vi "Digilens DLP Gen2 UI .vi"(11 "TopLevel In":refnum<class "TopLevel.lvclass">) -> (3 "TopLevel Out":refnum<class "TopLevel.lvclass">)   [LabVIEW 2022 SP3, in "TopLevel.lvclass"] (continued)
              disable-tunnel: ICP2-DO_Channel_Names."Recirc Pump On - R2" ("DO Channel") -> [w2353 w2369]
              disable-tunnel: w2344 -> [w2352 _]
              disable-tunnel: [w2351 w2354] -> w2343
              disable-tunnel: w2342 -> [w2350 w2370]
              disable-tunnel: "Recirc Pump On - R2" -> [w2349 w2356]
              disable-tunnel: w2340 -> [_ w2368]
              frame Disabled {
                n801 = call-dynamic "Set ICP2-DO Changed bit.vi"("error in (no error)"=w2350, "Value"=w2349, "DO Channel"=w2353, "IO in"=w2352) -> ("error out"=w2351:errorcluster)  [unwired: 6 in, 1 out]
              }
              frame Enabled {
                n802 = Format Into String(format string="%s", w2369) -> (resulting string=w2372:string)  [unwired: 2 in, 1 out]
                n803 = call "Set DO State (manual mode).vi"("error in (no error)"=w2370, "State"=w2356, "DO IOName"=w2372, "DAQ"=w2368) -> ("error out"=w2355:errorcluster, "DAQ"=w2357:refnum<class "DAQ.lvclass">)  [unwired: 6 in]
                n804 = Format Into String(format string="%s", error in=w2355, ICP2-DO_Channel_Names."SW_LED - Ink Valve - R2" ("DO Channel")) -> (resulting string=w2367:string, error out=w2364:errorcluster)  [unwired: 1 in]
                n805 = call "Set DO State (automation mode).vi"("error in (no error)"=w2364, "State"=w2356, "DO IOName"=w2367, "DAQ"=w2357) -> ("error out"=w2358:errorcluster, "DAQ"=w2360:refnum<class "DAQ.lvclass">)  [unwired: 6 in]
                n806 = Format Into String(format string="%s", error in=w2358, ICP2-DO_Channel_Names."Ink Flow Valve Open - R2" ("DO Channel")) -> (resulting string=w2361:string, error out=w2363:errorcluster)  [unwired: 1 in]
                n807 = call "Set DO State (automation mode).vi"("error in (no error)"=w2363, "State"=w2356, "DO IOName"=w2361, "DAQ"=w2360) -> ("error out"=w2354:errorcluster)  [unwired: 6 in, 1 out]
              }
            }
          }
          event "Recirc Pump On - R3": Value Change {
            n808 = event-data() -> ()  [unwired: 1 in, 6 out]
            n809 = Unbundle By Name(w2378) -> ("DAQ"=w2373:refnum<class "DAQ.lvclass">, "IO"=w2377:refnum<class "IO.lvclass">)
            n810 = disable-structure shown="Enabled" {
              disable-tunnel: ICP2-DO_Channel_Names."Recirc Pump On - R3" ("DO Channel") -> [w2386 w2401]
              disable-tunnel: w2377 -> [w2385 _]
              disable-tunnel: [w2384 w2387] -> w2376
              disable-tunnel: w2375 -> [w2383 w2403]
              disable-tunnel: "Recirc Pump On - R3" -> [w2382 w2389]
              disable-tunnel: w2373 -> [_ w2402]
              frame Disabled {
                n811 = call-dynamic "Set ICP2-DO Changed bit.vi"("error in (no error)"=w2383, "Value"=w2382, "DO Channel"=w2386, "IO in"=w2385) -> ("error out"=w2384:errorcluster)  [unwired: 6 in, 1 out]
              }
              frame Enabled {
                n812 = Format Into String(format string="%s", w2401) -> (resulting string=w2405:string)  [unwired: 2 in, 1 out]
                n813 = call "Set DO State (manual mode).vi"("error in (no error)"=w2403, "State"=w2389, "DO IOName"=w2405, "DAQ"=w2402) -> ("error out"=w2388:errorcluster, "DAQ"=w2390:refnum<class "DAQ.lvclass">)  [unwired: 6 in]
                n814 = Format Into String(format string="%s", error in=w2388, ICP2-DO_Channel_Names."SW_LED - Ink Valve - R3" ("DO Channel")) -> (resulting string=w2400:string, error out=w2397:errorcluster)  [unwired: 1 in]
                n815 = call "Set DO State (automation mode).vi"("error in (no error)"=w2397, "State"=w2389, "DO IOName"=w2400, "DAQ"=w2390) -> ("error out"=w2391:errorcluster, "DAQ"=w2393:refnum<class "DAQ.lvclass">)  [unwired: 6 in]
                n816 = Format Into String(format string="%s", error in=w2391, ICP2-DO_Channel_Names."Ink Flow Valve Open - R3" ("DO Channel")) -> (resulting string=w2394:string, error out=w2396:errorcluster)  [unwired: 1 in]
                n817 = call "Set DO State (automation mode).vi"("error in (no error)"=w2396, "State"=w2389, "DO IOName"=w2394, "DAQ"=w2393) -> ("error out"=w2387:errorcluster)  [unwired: 6 in, 1 out]
              }
            }
          }
          event "Recirc Pump On - R4": Value Change {
            n818 = event-data() -> ()  [unwired: 1 in, 6 out]
            n819 = Unbundle By Name(w2411) -> ("DAQ"=w2406:refnum<class "DAQ.lvclass">, "IO"=w2410:refnum<class "IO.lvclass">)
            n820 = disable-structure shown="Enabled" {
              disable-tunnel: ICP2-DO_Channel_Names."Recirc Pump On - R4" ("DO Channel") -> [w2419 w2434]
              disable-tunnel: w2410 -> [w2418 _]
              disable-tunnel: [w2417 w2420] -> w2409
              disable-tunnel: w2408 -> [w2416 w2436]
              disable-tunnel: "Recirc Pump On - R4" -> [w2415 w2421]
              disable-tunnel: w2406 -> [_ w2435]
              frame Disabled {
                n821 = call-dynamic "Set ICP2-DO Changed bit.vi"("error in (no error)"=w2416, "Value"=w2415, "DO Channel"=w2419, "IO in"=w2418) -> ("error out"=w2417:errorcluster)  [unwired: 6 in, 1 out]
              }
              frame Enabled {
                n822 = Format Into String(format string="%s", w2434) -> (resulting string=w2438:string)  [unwired: 2 in, 1 out]
                n823 = call "Set DO State (manual mode).vi"("error in (no error)"=w2436, "State"=w2421, "DO IOName"=w2438, "DAQ"=w2435) -> ("error out"=w2422:errorcluster, "DAQ"=w2423:refnum<class "DAQ.lvclass">)  [unwired: 6 in]
                n824 = Format Into String(format string="%s", error in=w2422, ICP2-DO_Channel_Names."SW_LED - Ink Valve - R4" ("DO Channel")) -> (resulting string=w2433:string, error out=w2430:errorcluster)  [unwired: 1 in]
                n825 = call "Set DO State (automation mode).vi"("error in (no error)"=w2430, "State"=w2421, "DO IOName"=w2433, "DAQ"=w2423) -> ("error out"=w2424:errorcluster, "DAQ"=w2426:refnum<class "DAQ.lvclass">)  [unwired: 6 in]
                n826 = Format Into String(format string="%s", error in=w2424, ICP2-DO_Channel_Names."Ink Flow Valve Open - R4" ("DO Channel")) -> (resulting string=w2427:string, error out=w2429:errorcluster)  [unwired: 1 in]
                n827 = call "Set DO State (automation mode).vi"("error in (no error)"=w2429, "State"=w2421, "DO IOName"=w2427, "DAQ"=w2426) -> ("error out"=w2420:errorcluster)  [unwired: 6 in, 1 out]
              }
            }
          }
          event "Recirc Pump On - R5": Value Change {
            n828 = event-data() -> ()  [unwired: 1 in, 6 out]
            n829 = Unbundle By Name(w2444) -> ("DAQ"=w2439:refnum<class "DAQ.lvclass">, "IO"=w2443:refnum<class "IO.lvclass">)
            n830 = disable-structure shown="Enabled" {
              disable-tunnel: ICP2-DO_Channel_Names."Recirc Pump On - R5" ("DO Channel") -> [w2452 w2468]
              disable-tunnel: w2443 -> [w2451 _]
              disable-tunnel: [w2450 w2453] -> w2442
              disable-tunnel: w2441 -> [w2449 w2469]
              disable-tunnel: "Recirc Pump On - R5" -> [w2448 w2455]
              disable-tunnel: w2439 -> [_ w2467]
              frame Disabled {
                n831 = call-dynamic "Set ICP2-DO Changed bit.vi"("error in (no error)"=w2449, "Value"=w2448, "DO Channel"=w2452, "IO in"=w2451) -> ("error out"=w2450:errorcluster)  [unwired: 6 in, 1 out]
              }
              frame Enabled {
                n832 = Format Into String(format string="%s", w2468) -> (resulting string=w2471:string)  [unwired: 2 in, 1 out]
                n833 = call "Set DO State (manual mode).vi"("error in (no error)"=w2469, "State"=w2455, "DO IOName"=w2471, "DAQ"=w2467) -> ("error out"=w2454:errorcluster, "DAQ"=w2456:refnum<class "DAQ.lvclass">)  [unwired: 6 in]
                n834 = Format Into String(format string="%s", error in=w2454, ICP2-DO_Channel_Names."SW_LED - Ink Valve - R5" ("DO Channel")) -> (resulting string=w2466:string, error out=w2463:errorcluster)  [unwired: 1 in]
                n835 = call "Set DO State (automation mode).vi"("error in (no error)"=w2463, "State"=w2455, "DO IOName"=w2466, "DAQ"=w2456) -> ("error out"=w2457:errorcluster, "DAQ"=w2459:refnum<class "DAQ.lvclass">)  [unwired: 6 in]
                n836 = Format Into String(format string="%s", error in=w2457, ICP2-DO_Channel_Names."Ink Flow Valve Open - R5" ("DO Channel")) -> (resulting string=w2460:string, error out=w2462:errorcluster)  [unwired: 1 in]
                n837 = call "Set DO State (automation mode).vi"("error in (no error)"=w2462, "State"=w2455, "DO IOName"=w2460, "DAQ"=w2459) -> ("error out"=w2453:errorcluster)  [unwired: 6 in, 1 out]
              }
            }
          }
          event "Recirc Pump On - R6": Value Change {
            n838 = event-data() -> ()  [unwired: 1 in, 6 out]
            n839 = Unbundle By Name(w2477) -> ("DAQ"=w2472:refnum<class "DAQ.lvclass">, "IO"=w2476:refnum<class "IO.lvclass">)
            n840 = disable-structure shown="Enabled" {
              disable-tunnel: ICP2-DO_Channel_Names."Recirc Pump On - R6" ("DO Channel") -> [w2485 w2500]
              disable-tunnel: w2476 -> [w2484 _]
              disable-tunnel: [w2483 w2487] -> w2475
              disable-tunnel: w2474 -> [w2482 w2502]
              disable-tunnel: "Recirc Pump On - R6" -> [w2481 w2486]
              disable-tunnel: w2472 -> [_ w2501]
              frame Disabled {
                n841 = call-dynamic "Set ICP2-DO Changed bit.vi"("error in (no error)"=w2482, "Value"=w2481, "DO Channel"=w2485, "IO in"=w2484) -> ("error out"=w2483:errorcluster)  [unwired: 6 in, 1 out]
              }
              frame Enabled {
                n842 = Format Into String(format string="%s", w2500) -> (resulting string=w2504:string)  [unwired: 2 in, 1 out]
                n843 = call "Set DO State (manual mode).vi"("error in (no error)"=w2502, "State"=w2486, "DO IOName"=w2504, "DAQ"=w2501) -> ("error out"=w2488:errorcluster, "DAQ"=w2489:refnum<class "DAQ.lvclass">)  [unwired: 6 in]
                n844 = Format Into String(format string="%s", error in=w2488, ICP2-DO_Channel_Names."SW_LED - Ink Valve - R6" ("DO Channel")) -> (resulting string=w2499:string, error out=w2496:errorcluster)  [unwired: 1 in]
                n845 = call "Set DO State (automation mode).vi"("error in (no error)"=w2496, "State"=w2486, "DO IOName"=w2499, "DAQ"=w2489) -> ("error out"=w2490:errorcluster, "DAQ"=w2492:refnum<class "DAQ.lvclass">)  [unwired: 6 in]
                n846 = Format Into String(format string="%s", error in=w2490, ICP2-DO_Channel_Names."Ink Flow Valve Open - R6" ("DO Channel")) -> (resulting string=w2493:string, error out=w2495:errorcluster)  [unwired: 1 in]
                n847 = call "Set DO State (automation mode).vi"("error in (no error)"=w2495, "State"=w2486, "DO IOName"=w2493, "DAQ"=w2492) -> ("error out"=w2487:errorcluster)  [unwired: 6 in, 1 out]
              }
            }
          }
          event "Meniscus Pressure Reg PWR - R1": Value Change {
            n848 = event-data() -> ()  [unwired: 1 in, 6 out]
            n849 = Unbundle By Name(w2510) -> ("DAQ"=w2505:refnum<class "DAQ.lvclass">, "IO"=w2509:refnum<class "IO.lvclass">)
            n850 = disable-structure shown="Enabled" {
              disable-tunnel: ICP1-D0_Channel_Names."Meniscus Pressure Reg PWR - R1" ("DO Channel") -> [w2518 w2520]
              disable-tunnel: w2509 -> [w2517 _]
              disable-tunnel: [w2516 w2522] -> w2508
              disable-tunnel: w2507 -> [w2515 w2523]
              disable-tunnel: "Meniscus Pressure Reg PWR - R1" -> [w2514 w2521]
              disable-tunnel: w2505 -> [_ w2519]
              frame Disabled {
                n851 = call-dynamic "Set ICP1-DO Changed bit.vi"("error in (no error)"=w2515, "Value"=w2514, "DO Channel"=w2518, "IO in"=w2517) -> ("error out"=w2516:errorcluster)  [unwired: 6 in, 1 out]
              }
              frame Enabled {
                n852 = Format Into String(format string="%s", w2520) -> (resulting string=w2525:string)  [unwired: 2 in, 1 out]
                n853 = call "Set DO State (manual mode).vi"("error in (no error)"=w2523, "State"=w2521, "DO IOName"=w2525, "DAQ"=w2519) -> ("error out"=w2522:errorcluster)  [unwired: 6 in, 1 out]
              }
            }
          }
          event "Meniscus Pressure Reg PWR - R2": Value Change {
            n854 = event-data() -> ()  [unwired: 1 in, 6 out]
            n855 = Unbundle By Name(w2531) -> ("DAQ"=w2526:refnum<class "DAQ.lvclass">, "IO"=w2530:refnum<class "IO.lvclass">)
            n856 = disable-structure shown="Enabled" {
              disable-tunnel: ICP1-D0_Channel_Names."Meniscus Pressure Reg PWR - R2" ("DO Channel") -> [w2539 w2542]
              disable-tunnel: w2530 -> [w2538 _]
              disable-tunnel: [w2537 w2540] -> w2529
              disable-tunnel: w2528 -> [w2536 w2541]
              disable-tunnel: "Meniscus Pressure Reg PWR - R2" -> [w2535 w2544]
              disable-tunnel: w2526 -> [_ w2543]
              frame Disabled {
                n857 = call-dynamic "Set ICP1-DO Changed bit.vi"("error in (no error)"=w2536, "Value"=w2535, "DO Channel"=w2539, "IO in"=w2538) -> ("error out"=w2537:errorcluster)  [unwired: 6 in, 1 out]
              }
              frame Enabled {
                n858 = Format Into String(format string="%s", w2542) -> (resulting string=w2546:string)  [unwired: 2 in, 1 out]
                n859 = call "Set DO State (manual mode).vi"("error in (no error)"=w2541, "State"=w2544, "DO IOName"=w2546, "DAQ"=w2543) -> ("error out"=w2540:errorcluster)  [unwired: 6 in, 1 out]
              }
            }
          }
          event "Meniscus Pressure Reg PWR - R3": Value Change {
            n860 = event-data() -> ()  [unwired: 1 in, 6 out]
            n861 = Unbundle By Name(w2552) -> ("DAQ"=w2547:refnum<class "DAQ.lvclass">, "IO"=w2551:refnum<class "IO.lvclass">)
            n862 = disable-structure shown="Enabled" {
              disable-tunnel: ICP1-D0_Channel_Names."Meniscus Pressure Reg PWR - R3" ("DO Channel") -> [w2560 w2561]
              disable-tunnel: w2551 -> [w2559 _]
              disable-tunnel: [w2558 w2563] -> w2550
              disable-tunnel: w2549 -> [w2557 w2564]
              disable-tunnel: "Meniscus Pressure Reg PWR - R3" -> [w2556 w2565]
              disable-tunnel: w2547 -> [_ w2562]
              frame Disabled {
                n863 = call-dynamic "Set ICP1-DO Changed bit.vi"("error in (no error)"=w2557, "Value"=w2556, "DO Channel"=w2560, "IO in"=w2559) -> ("error out"=w2558:errorcluster)  [unwired: 6 in, 1 out]
              }
              frame Enabled {
                n864 = Format Into String(format string="%s", w2561) -> (resulting string=w2567:string)  [unwired: 2 in, 1 out]
                n865 = call "Set DO State (manual mode).vi"("error in (no error)"=w2564, "State"=w2565, "DO IOName"=w2567, "DAQ"=w2562) -> ("error out"=w2563:errorcluster)  [unwired: 6 in, 1 out]
              }
            }
          }
          event "Meniscus Pressure Reg PWR - R4": Value Change {
            n866 = event-data() -> ()  [unwired: 1 in, 6 out]
            n867 = Unbundle By Name(w2573) -> ("DAQ"=w2568:refnum<class "DAQ.lvclass">, "IO"=w2572:refnum<class "IO.lvclass">)
            n868 = disable-structure shown="Enabled" {
              disable-tunnel: ICP1-D0_Channel_Names."Meniscus Pressure Reg PWR - R4" ("DO Channel") -> [w2581 w2583]
              disable-tunnel: w2572 -> [w2580 _]
              disable-tunnel: [w2579 w2585] -> w2571
              disable-tunnel: w2570 -> [w2578 w2586]
              disable-tunnel: "Meniscus Pressure Reg PWR - R4" -> [w2577 w2584]
              disable-tunnel: w2568 -> [_ w2582]
              frame Disabled {
                n869 = call-dynamic "Set ICP1-DO Changed bit.vi"("error in (no error)"=w2578, "Value"=w2577, "DO Channel"=w2581, "IO in"=w2580) -> ("error out"=w2579:errorcluster)  [unwired: 6 in, 1 out]
              }
              frame Enabled {
                n870 = Format Into String(format string="%s", w2583) -> (resulting string=w2588:string)  [unwired: 2 in, 1 out]
                n871 = call "Set DO State (manual mode).vi"("error in (no error)"=w2586, "State"=w2584, "DO IOName"=w2588, "DAQ"=w2582) -> ("error out"=w2585:errorcluster)  [unwired: 6 in, 1 out]
              }
            }
          }
          event "Meniscus Pressure Reg PWR - R5": Value Change {
            n872 = event-data() -> ()  [unwired: 1 in, 6 out]
            n873 = Unbundle By Name(w2594) -> ("DAQ"=w2589:refnum<class "DAQ.lvclass">, "IO"=w2593:refnum<class "IO.lvclass">)
            n874 = disable-structure shown="Enabled" {
              disable-tunnel: ICP1-D0_Channel_Names."Meniscus Pressure Reg PWR - R5" ("DO Channel") -> [w2602 w2603]
              disable-tunnel: w2593 -> [w2601 _]
              disable-tunnel: [w2600 w2605] -> w2592
              disable-tunnel: w2591 -> [w2599 w2606]
              disable-tunnel: "Meniscus Pressure Reg PWR - R5" -> [w2598 w2607]
              disable-tunnel: w2589 -> [_ w2604]
              frame Disabled {
                n875 = call-dynamic "Set ICP1-DO Changed bit.vi"("error in (no error)"=w2599, "Value"=w2598, "DO Channel"=w2602, "IO in"=w2601) -> ("error out"=w2600:errorcluster)  [unwired: 6 in, 1 out]
              }
              frame Enabled {
                n876 = Format Into String(format string="%s", w2603) -> (resulting string=w2609:string)  [unwired: 2 in, 1 out]
                n877 = call "Set DO State (manual mode).vi"("error in (no error)"=w2606, "State"=w2607, "DO IOName"=w2609, "DAQ"=w2604) -> ("error out"=w2605:errorcluster)  [unwired: 6 in, 1 out]
              }
            }
          }
          event "Meniscus Pressure Reg PWR - R6": Value Change {
            n878 = event-data() -> ()  [unwired: 1 in, 6 out]
            n879 = Unbundle By Name(w2615) -> ("DAQ"=w2610:refnum<class "DAQ.lvclass">, "IO"=w2614:refnum<class "IO.lvclass">)
            n880 = disable-structure shown="Enabled" {
              disable-tunnel: ICP1-D0_Channel_Names."Meniscus Pressure Reg PWR - R6" ("DO Channel") -> [w2623 w2624]
              disable-tunnel: w2614 -> [w2622 _]
              disable-tunnel: [w2621 w2627] -> w2613
              disable-tunnel: w2612 -> [w2620 w2628]
              disable-tunnel: "Meniscus Pressure Reg PWR - R6" -> [w2619 w2626]
              disable-tunnel: w2610 -> [_ w2625]
              frame Disabled {
                n881 = call-dynamic "Set ICP1-DO Changed bit.vi"("error in (no error)"=w2620, "Value"=w2619, "DO Channel"=w2623, "IO in"=w2622) -> ("error out"=w2621:errorcluster)  [unwired: 6 in, 1 out]
              }
              frame Enabled {
                n882 = Format Into String(format string="%s", w2624) -> (resulting string=w2630:string)  [unwired: 2 in, 1 out]
                n883 = call "Set DO State (manual mode).vi"("error in (no error)"=w2628, "State"=w2626, "DO IOName"=w2630, "DAQ"=w2625) -> ("error out"=w2627:errorcluster)  [unwired: 6 in, 1 out]
              }
            }
          }
          event "ClearStageAlarm": Value Change {
            n884 = event-data() -> ()  [unwired: 1 in, 6 out]
            n885 = Unbundle By Name(w2662) -> ("Motor Controller"=w2641:refnum<class "Motor Controller.lvclass">, "IO"=w2653:refnum<class "IO.lvclass">, "DAQ"=w2636:refnum<class "DAQ.lvclass">)
            n886 = call "API_AbortStage.vi"("Wait (F)"=FALSE, "error in (no error)"=w2640, "Task ID"="AbortMotor", "Motor Controller in"=w2641) -> ("error out"=w2639:errorcluster)  [unwired: 5 in, 2 out]
            n887 = disable-structure shown="Enabled" {
              disable-tunnel: w2653 -> [w2715 w2724]
              disable-tunnel: [w2714 w2724] -> w2652
              disable-tunnel: [w2713 w2720] -> w2648
              disable-tunnel: w2639 -> [w2712 w2721]
              disable-tunnel: ICP1-D0_Channel_Names."Servo ON" ("DO Channel") -> [w2711 w2718]
              disable-tunnel: FALSE -> [w2710 w2717]
              disable-tunnel: w2636 -> [w2709 w2719]
              disable-tunnel: [w2709 w2716] -> w2635
              frame Disabled {
                n888 = call-dynamic "Set ICP1-DO Changed bit.vi"("error in (no error)"=w2712, "Value"=w2710, "DO Channel"=w2711, "IO in"=w2715) -> ("error out"=w2713:errorcluster, "IO out"=w2714:refnum<class "IO.lvclass">)  [unwired: 6 in]
              }
              frame Enabled {
                n889 = Format Into String(format string="%s", w2718) -> (resulting string=w2723:string)  [unwired: 2 in, 1 out]
                n890 = call "Set DO State (manual mode).vi"("error in (no error)"=w2721, "State"=w2717, "DO IOName"=w2723, "DAQ"=w2719) -> ("error out"=w2720:errorcluster, "DAQ"=w2716:refnum<class "DAQ.lvclass">)  [unwired: 6 in]
              }
            }
            n891 = call <userlib>:"Wait (ms)__ogtk.vi"("error in (no error)"=w2648, "milliseconds to wait"=u32 100) -> ("error out"=w2647:errorcluster)  [unwired: 8 in, 1 out]
            n892 = disable-structure shown="Enabled" {
              disable-tunnel: ICP1-D0_Channel_Names."Clear Stage Alarm" ("DO Channel") -> [w2687 w2689]
              disable-tunnel: TRUE -> [w2686 w2691]
              disable-tunnel: [w2685 w2696] -> w2658
              disable-tunnel: [w2684 w2692] -> w2655
              disable-tunnel: w2652 -> [w2683 w2696]
              disable-tunnel: w2647 -> [w2681 w2693]
              disable-tunnel: w2635 -> [_ w2690]
              disable-tunnel: [_ w2688] -> w2634
              frame Disabled {
                n893 = call-dynamic "Set ICP1-DO Changed bit.vi"("Wait (F)"=TRUE, "error in (no error)"=w2681, "Value"=w2686, "DO Channel"=w2687, "IO in"=w2683) -> ("error out"=w2684:errorcluster, "IO out"=w2685:refnum<class "IO.lvclass">)  [unwired: 5 in]
              }
              frame Enabled {
                n894 = Format Into String(format string="%s", w2689) -> (resulting string=w2695:string)  [unwired: 2 in, 1 out]
                n895 = call "Set DO State (manual mode).vi"("error in (no error)"=w2693, "State"=w2691, "DO IOName"=w2695, "DAQ"=w2690) -> ("error out"=w2692:errorcluster, "DAQ"=w2688:refnum<class "DAQ.lvclass">)  [unwired: 6 in]
              }
            }
            n896 = local write "ClearStageAlarm"(FALSE ("ClearStageAlarm")) -> ()
            n897 = call <userlib>:"Wait (ms)__ogtk.vi"("error in (no error)"=w2655, "milliseconds to wait"=u32 300) -> ("error out"=w2657:errorcluster)  [unwired: 8 in, 1 out]
            n898 = disable-structure shown="Enabled" {
              disable-tunnel: ICP1-D0_Channel_Names."Clear Stage Alarm" ("DO Channel") -> [w2671 w2673]
              disable-tunnel: w2658 -> [w2670 w2680]
              disable-tunnel: w2657 -> [w2669 w2676]
              disable-tunnel: FALSE -> [w2668 w2675]
              disable-tunnel: [w2667 w2680] -> w2651
              disable-tunnel: [w2666 w2677] -> w2650
              disable-tunnel: w2634 -> [_ w2674]
              disable-tunnel: [_ w2672] -> w2633
              frame Disabled {
                n899 = call-dynamic "Set ICP1-DO Changed bit.vi"("error in (no error)"=w2669, "Value"=w2668, "DO Channel"=w2671, "IO in"=w2670) -> ("error out"=w2666:errorcluster, "IO out"=w2667:refnum<class "IO.lvclass">)  [unwired: 6 in]
              }
              frame Enabled {
                n900 = Format Into String(format string="%s", w2673) -> (resulting string=w2679:string)  [unwired: 2 in, 1 out]
                n901 = call "Set DO State (manual mode).vi"("error in (no error)"=w2676, "State"=w2675, "DO IOName"=w2679, "DAQ"=w2674) -> ("error out"=w2677:errorcluster, "DAQ"=w2672:refnum<class "DAQ.lvclass">)  [unwired: 6 in]
              }
            }
            n902 = call <userlib>:"Wait (ms)__ogtk.vi"("error in (no error)"=w2650, "milliseconds to wait"=u32 100) -> ("error out"=w2645:errorcluster)  [unwired: 8 in, 1 out]
            n903 = disable-structure shown="Enabled" {
              disable-tunnel: w2651 -> [w2701 _]
              disable-tunnel: w2645 -> [w2700 w2706]
              disable-tunnel: [w2699 w2705] -> w2649
              disable-tunnel: w2633 -> [_ w2704]
              disable-tunnel: ICP1-D0_Channel_Names."Servo ON" ("DO Channel") -> [w2698 w2702]
              disable-tunnel: TRUE -> [w2697 w2703]
              frame Disabled {
                n904 = call-dynamic "Set ICP1-DO Changed bit.vi"("error in (no error)"=w2700, "Value"=w2697, "DO Channel"=w2698, "IO in"=w2701) -> ("error out"=w2699:errorcluster)  [unwired: 6 in, 1 out]
              }
              frame Enabled {
                n905 = Format Into String(format string="%s", w2702) -> (resulting string=w2708:string)  [unwired: 2 in, 1 out]
                n906 = call "Set DO State (manual mode).vi"("error in (no error)"=w2706, "State"=w2703, "DO IOName"=w2708, "DAQ"=w2704) -> ("error out"=w2705:errorcluster)  [unwired: 6 in, 1 out]
              }
            }
          }
          event Value Change {
            n907 = event-data() -> ("NewVal"=w2726:T1)  [unwired: 1 in, 5 out]
            n908 = Unbundle By Name(w2731) -> ("DAQ"=w2725:refnum<class "DAQ.lvclass">, "IO"=w2729:refnum<class "IO.lvclass">)
            n909 = disable-structure shown="Enabled" {
              disable-tunnel: ICP1-D0_Channel_Names."Servo ON" ("DO Channel") -> [w2738 w2739]
              disable-tunnel: w2729 -> [w2737 _]
              disable-tunnel: [w2736 w2742] -> w2728
              disable-tunnel: w2727 -> [w2735 w2743]
              disable-tunnel: w2726 -> [w2734 w2741]
              disable-tunnel: w2725 -> [_ w2740]
              frame Disabled {
                n910 = call-dynamic "Set ICP1-DO Changed bit.vi"("error in (no error)"=w2735, "Value"=w2734, "DO Channel"=w2738, "IO in"=w2737) -> ("error out"=w2736:errorcluster)  [unwired: 6 in, 1 out]
              }
              frame Enabled {
                n911 = Format Into String(format string="%s", w2739) -> (resulting string=w2745:string)  [unwired: 2 in, 1 out]
                n912 = call "Set DO State (manual mode).vi"("error in (no error)"=w2743, "State"=w2741, "DO IOName"=w2745, "DAQ"=w2740) -> ("error out"=w2742:errorcluster)  [unwired: 6 in, 1 out]
              }
            }
          }
          event "Purge Valve Open - R1": Value Change {
            n913 = event-data() -> ()  [unwired: 1 in, 6 out]
            n914 = Unbundle By Name(w2751) -> ("DAQ"=w2746:refnum<class "DAQ.lvclass">, "IO"=w2750:refnum<class "IO.lvclass">)
            n915 = disable-structure shown="Enabled" {
              disable-tunnel: ICP1-D0_Channel_Names."Purge Valve Open - R1" ("DO Channel") -> [w2759 w2761]
              disable-tunnel: w2750 -> [w2758 _]
              disable-tunnel: [w2757 w2763] -> w2749
              disable-tunnel: w2748 -> [w2756 w2764]
              disable-tunnel: "Purge Valve Open - R1" -> [w2755 w2762]
              disable-tunnel: w2746 -> [_ w2760]
              frame Disabled {
                n916 = call-dynamic "Set ICP1-DO Changed bit.vi"("error in (no error)"=w2756, "Value"=w2755, "DO Channel"=w2759, "IO in"=w2758) -> ("error out"=w2757:errorcluster)  [unwired: 6 in, 1 out]
              }
              frame Enabled {
                n917 = Format Into String(format string="%s", w2761) -> (resulting string=w2766:string)  [unwired: 2 in, 1 out]
                n918 = call "Set DO State (manual mode).vi"("error in (no error)"=w2764, "State"=w2762, "DO IOName"=w2766, "DAQ"=w2760) -> ("error out"=w2763:errorcluster)  [unwired: 6 in, 1 out]
              }
            }
          }
          event "Purge Valve Open - R2": Value Change {
            n919 = event-data() -> ()  [unwired: 1 in, 6 out]
            n920 = Unbundle By Name(w2772) -> ("DAQ"=w2767:refnum<class "DAQ.lvclass">, "IO"=w2771:refnum<class "IO.lvclass">)
            n921 = disable-structure shown="Enabled" {
              disable-tunnel: ICP1-D0_Channel_Names."Purge Valve Open - R2" ("DO Channel") -> [w2780 w2782]
              disable-tunnel: w2771 -> [w2779 _]
              disable-tunnel: [w2778 w2784] -> w2770
              disable-tunnel: w2769 -> [w2777 w2785]
              disable-tunnel: "Purge Valve Open - R2" -> [w2776 w2783]
              disable-tunnel: w2767 -> [_ w2781]
              frame Disabled {
                n922 = call-dynamic "Set ICP1-DO Changed bit.vi"("error in (no error)"=w2777, "Value"=w2776, "DO Channel"=w2780, "IO in"=w2779) -> ("error out"=w2778:errorcluster)  [unwired: 6 in, 1 out]
              }
              frame Enabled {
                n923 = Format Into String(format string="%s", w2782) -> (resulting string=w2787:string)  [unwired: 2 in, 1 out]
                n924 = call "Set DO State (manual mode).vi"("error in (no error)"=w2785, "State"=w2783, "DO IOName"=w2787, "DAQ"=w2781) -> ("error out"=w2784:errorcluster)  [unwired: 6 in, 1 out]
              }
            }
          }
          event "Purge Valve Open - R3": Value Change {
            n925 = event-data() -> ()  [unwired: 1 in, 6 out]
            n926 = Unbundle By Name(w2793) -> ("DAQ"=w2788:refnum<class "DAQ.lvclass">, "IO"=w2792:refnum<class "IO.lvclass">)
            n927 = disable-structure shown="Enabled" {
              disable-tunnel: ICP1-D0_Channel_Names."Purge Valve Open - R3" ("DO Channel") -> [w2801 w2803]
              disable-tunnel: w2792 -> [w2800 _]
              disable-tunnel: [w2799 w2804] -> w2791
              disable-tunnel: w2790 -> [w2798 w2805]
              disable-tunnel: "Purge Valve Open - R3" -> [w2797 w2806]
              disable-tunnel: w2788 -> [_ w2802]
              frame Disabled {
                n928 = call-dynamic "Set ICP1-DO Changed bit.vi"("error in (no error)"=w2798, "Value"=w2797, "DO Channel"=w2801, "IO in"=w2800) -> ("error out"=w2799:errorcluster)  [unwired: 6 in, 1 out]
              }
              frame Enabled {
                n929 = Format Into String(format string="%s", w2803) -> (resulting string=w2808:string)  [unwired: 2 in, 1 out]
                n930 = call "Set DO State (manual mode).vi"("error in (no error)"=w2805, "State"=w2806, "DO IOName"=w2808, "DAQ"=w2802) -> ("error out"=w2804:errorcluster)  [unwired: 6 in, 1 out]
              }
            }
          }
          event "Purge Valve Open - R4": Value Change {
            n931 = event-data() -> ()  [unwired: 1 in, 6 out]
            n932 = Unbundle By Name(w2814) -> ("DAQ"=w2809:refnum<class "DAQ.lvclass">, "IO"=w2813:refnum<class "IO.lvclass">)
            n933 = disable-structure shown="Enabled" {
              disable-tunnel: ICP1-D0_Channel_Names."Purge Valve Open - R4" ("DO Channel") -> [w2822 w2823]
              disable-tunnel: w2813 -> [w2821 _]
              disable-tunnel: [w2820 w2825] -> w2812
              disable-tunnel: w2811 -> [w2819 w2826]
              disable-tunnel: "Purge Valve Open - R4" -> [w2818 w2827]
              disable-tunnel: w2809 -> [_ w2824]
              frame Disabled {
                n934 = call-dynamic "Set ICP1-DO Changed bit.vi"("error in (no error)"=w2819, "Value"=w2818, "DO Channel"=w2822, "IO in"=w2821) -> ("error out"=w2820:errorcluster)  [unwired: 6 in, 1 out]
              }
              frame Enabled {
                n935 = Format Into String(format string="%s", w2823) -> (resulting string=w2829:string)  [unwired: 2 in, 1 out]
                n936 = call "Set DO State (manual mode).vi"("error in (no error)"=w2826, "State"=w2827, "DO IOName"=w2829, "DAQ"=w2824) -> ("error out"=w2825:errorcluster)  [unwired: 6 in, 1 out]
              }
            }
          }
          event "Purge Valve Open - R5": Value Change {
            n937 = event-data() -> ()  [unwired: 1 in, 6 out]
            n938 = Unbundle By Name(w2835) -> ("DAQ"=w2830:refnum<class "DAQ.lvclass">, "IO"=w2834:refnum<class "IO.lvclass">)
            n939 = disable-structure shown="Enabled" {
              disable-tunnel: ICP1-D0_Channel_Names."Purge Valve Open - R5" ("DO Channel") -> [w2843 w2845]
              disable-tunnel: w2834 -> [w2842 _]
              disable-tunnel: [w2841 w2846] -> w2833
              disable-tunnel: w2832 -> [w2840 w2847]
              disable-tunnel: "Purge Valve Open - R5" -> [w2839 w2848]
              disable-tunnel: w2830 -> [_ w2844]
              frame Disabled {
                n940 = call-dynamic "Set ICP1-DO Changed bit.vi"("error in (no error)"=w2840, "Value"=w2839, "DO Channel"=w2843, "IO in"=w2842) -> ("error out"=w2841:errorcluster)  [unwired: 6 in, 1 out]
              }
              frame Enabled {
                n941 = Format Into String(format string="%s", w2845) -> (resulting string=w2850:string)  [unwired: 2 in, 1 out]
                n942 = call "Set DO State (manual mode).vi"("error in (no error)"=w2847, "State"=w2848, "DO IOName"=w2850, "DAQ"=w2844) -> ("error out"=w2846:errorcluster)  [unwired: 6 in, 1 out]
              }
            }
          }
          event "Purge Valve Open - R6": Value Change {
            n943 = event-data() -> ()  [unwired: 1 in, 6 out]
            n944 = Unbundle By Name(w2856) -> ("DAQ"=w2851:refnum<class "DAQ.lvclass">, "IO"=w2855:refnum<class "IO.lvclass">)
            n945 = disable-structure shown="Enabled" {
              disable-tunnel: ICP1-D0_Channel_Names."Purge Valve Open - R6" ("DO Channel") -> [w2864 w2866]
              disable-tunnel: w2855 -> [w2863 _]
              disable-tunnel: [w2862 w2868] -> w2854
              disable-tunnel: w2853 -> [w2861 w2869]
              disable-tunnel: "Purge Valve Open - R6" -> [w2860 w2867]
              disable-tunnel: w2851 -> [_ w2865]
              frame Disabled {
                n946 = call-dynamic "Set ICP1-DO Changed bit.vi"("error in (no error)"=w2861, "Value"=w2860, "DO Channel"=w2864, "IO in"=w2863) -> ("error out"=w2862:errorcluster)  [unwired: 6 in, 1 out]
              }
              frame Enabled {
                n947 = Format Into String(format string="%s", w2866) -> (resulting string=w2871:string)  [unwired: 2 in, 1 out]
                n948 = call "Set DO State (manual mode).vi"("error in (no error)"=w2869, "State"=w2867, "DO IOName"=w2871, "DAQ"=w2865) -> ("error out"=w2868:errorcluster)  [unwired: 6 in, 1 out]
              }
            }
          }
          event "Meniscus Pressure Set - R1-Set", "Meniscus Pressure Set - R2-Set", "Meniscus Pressure Set - R3-Set", "Meniscus Pressure Set - R4-Set", "Meniscus Pressure Set - R5-Set", "Meniscus Pressure Set - R6-Set": Value Change {
            n949 = event-data() -> ("CtlRef"=w2873:refnum<vi>)  [unwired: 1 in, 5 out]
            n950 = property class="Bool"(reference=w2873) -> ("Label.Text"=w2874:string)  [unwired: 1 in, 2 out]
            n951 = case shown="Default" w2874 {
              tunnel: ["" ("State(s) in Front (\"\")") "Set Meniscus Pressure>>R1" ("State(s) in Front (\"\")") "Set Meniscus Pressure>>R2" ("State(s) in Front (\"\")") "Set Meniscus Pressure>>R3" ("State(s) in Front (\"\")") "Set Meniscus Pressure>>R4" ("State(s) in Front (\"\")") "Set Meniscus Pressure>>R5" ("State(s) in Front (\"\")") "Set Meniscus Pressure>>R6" ("State(s) in Front (\"\")")] -> w2872
              frame Default {
              }
              frame "Meniscus Pressure Set - R1-Set " {
              }
              frame "Meniscus Pressure Set - R2-Set" {
              }
              frame "Meniscus Pressure Set - R3-Set" {
              }
              frame "Meniscus Pressure Set - R4-Set" {
              }
              frame "Meniscus Pressure Set - R5-Set" {
              }
              frame "Meniscus Pressure Set - R6-Set" {
              }
            }
            n952 = call <vilib>:"Add State(s) to Queue__JKI_lib_State_Machine.vi"("State(s) in Front (\"\")"=w2872, "State(s) in (\"\")"=w2875) -> ("States Out"=w2876:string)  [unwired: 13 in]
          }
          event "Meniscus Pressure Set - R1", "Meniscus Pressure Set - R2", "Meniscus Pressure Set - R3", "Meniscus Pressure Set - R4", "Meniscus Pressure Set - R5", "Meniscus Pressure Set - R6": Key Down {
            n953 = event-data() -> ("CtlRef"=w2890:refnum<vi>, "VKey"=w2891:T79)  [unwired: 1 in, 8 out]
            n954 = case shown="\"Return\"" w2891 {
              tunnel: w2890 -> [_ w2903]
              tunnel: w2888 -> [w2896 w2901]
              tunnel: [w2896 w2900] -> w2889
              tunnel: [_ w2898] -> w2887
              frame "ASCII", Default {
              }
              frame "Return" {
                n955 = property class="DigNum (strict)" props=["Key Focus", "Value", "Key Focus", "Label", "Text"](reference=w2903, error in=w2901, "Key Focus"=FALSE, "Key Focus"=TRUE) -> (error out=w2900:errorcluster, "Label.Text"=w2899:string)  [unwired: 2 out]
                n956 = case shown="\"Meniscus Pressure Set - R1\"" w2899 {
                  tunnel: [_ "Set Meniscus Pressure>>R1" ("State(s) in Front (\"\")") "Set Meniscus Pressure>>R2" ("State(s) in Front (\"\")") "Set Meniscus Pressure>>R3" ("State(s) in Front (\"\")") "Set Meniscus Pressure>>R4" ("State(s) in Front (\"\")") "Set Meniscus Pressure>>R5" ("State(s) in Front (\"\")") "Set Meniscus Pressure>>R6" ("State(s) in Front (\"\")")] -> w2898
                  frame Default {
                  }
                  frame "Meniscus Pressure Set - R1" {
                  }
                  frame "Meniscus Pressure Set - R2" {
                  }
                  frame "Meniscus Pressure Set - R3" {
                  }
                  frame "Meniscus Pressure Set - R4" {
                  }
                  frame "Meniscus Pressure Set - R5" {
                  }
                  frame "Meniscus Pressure Set - R6" {
                  }
                }
              }
            }
            n957 = call <vilib>:"Add State(s) to Queue__JKI_lib_State_Machine.vi"("State(s) in Front (\"\")"=w2887, "State(s) in (\"\")"=w2893) -> ("States Out"=w2892:string)  [unwired: 13 in]
          }
          event "Meniscus Pressure Set - R1": Value Change {
            n958 = event-data() -> ()  [unwired: 1 in, 6 out]
            n959 = disable-structure shown="Disabled" {
              disable-tunnel: ["Set Meniscus Pressure>>R1" ("State(s) in Front (\"\")") _] -> w2910
              frame Disabled {
              }
              frame Enabled {
              }
            }
            n960 = call <vilib>:"Add State(s) to Queue__JKI_lib_State_Machine.vi"("State(s) in Front (\"\")"=w2910, "State(s) in (\"\")"=w2912) -> ("States Out"=w2911:string)  [unwired: 13 in]
          }
          event "Meniscus Pressure Set - R2": Value Change {
            n961 = event-data() -> ()  [unwired: 1 in, 6 out]
            n962 = disable-structure shown="Disabled" {
              disable-tunnel: ["Set Meniscus Pressure>>R2" ("State(s) in Front (\"\")") _] -> w2917
              frame Disabled {
              }
              frame Enabled {
              }
            }
            n963 = call <vilib>:"Add State(s) to Queue__JKI_lib_State_Machine.vi"("State(s) in Front (\"\")"=w2917, "State(s) in (\"\")"=w2919) -> ("States Out"=w2918:string)  [unwired: 13 in]
          }
          event "Meniscus Pressure Set - R3": Value Change {
            n964 = event-data() -> ()  [unwired: 1 in, 6 out]
            n965 = disable-structure shown="Disabled" {
              disable-tunnel: ["Set Meniscus Pressure>>R3" ("State(s) in Front (\"\")") _] -> w2924
              frame Disabled {
              }
              frame Enabled {
              }
            }
            n966 = call <vilib>:"Add State(s) to Queue__JKI_lib_State_Machine.vi"("State(s) in Front (\"\")"=w2924, "State(s) in (\"\")"=w2926) -> ("States Out"=w2925:string)  [unwired: 13 in]
          }
          event "Meniscus Pressure Set - R4": Value Change {
            n967 = event-data() -> ()  [unwired: 1 in, 6 out]
            n968 = disable-structure shown="Disabled" {
              disable-tunnel: ["Set Meniscus Pressure>>R4" ("State(s) in Front (\"\")") _] -> w2931
              frame Disabled {
              }
              frame Enabled {
              }
            }
            n969 = call <vilib>:"Add State(s) to Queue__JKI_lib_State_Machine.vi"("State(s) in Front (\"\")"=w2931, "State(s) in (\"\")"=w2933) -> ("States Out"=w2932:string)  [unwired: 13 in]
          }
          event "Meniscus Pressure Set - R5": Value Change {
            n970 = event-data() -> ()  [unwired: 1 in, 6 out]
            n971 = disable-structure shown="Disabled" {
              disable-tunnel: ["Set Meniscus Pressure>>R5" ("State(s) in Front (\"\")") _] -> w2938
              frame Disabled {
              }
              frame Enabled {
              }
            }
            n972 = call <vilib>:"Add State(s) to Queue__JKI_lib_State_Machine.vi"("State(s) in Front (\"\")"=w2938, "State(s) in (\"\")"=w2940) -> ("States Out"=w2939:string)  [unwired: 13 in]
          }
          event "Meniscus Pressure Set - R6": Value Change {
            n973 = event-data() -> ()  [unwired: 1 in, 6 out]
            n974 = disable-structure shown="Disabled" {
              disable-tunnel: ["Set Meniscus Pressure>>R6" ("State(s) in Front (\"\")") _] -> w2945
              frame Disabled {
              }
              frame Enabled {
              }
            }
            n975 = call <vilib>:"Add State(s) to Queue__JKI_lib_State_Machine.vi"("State(s) in Front (\"\")"=w2945, "State(s) in (\"\")"=w2947) -> ("States Out"=w2946:string)  [unwired: 13 in]
          }
          event "Meniscus Vac Pump Speed-Set": Value Change {
            n976 = event-data() -> ()  [unwired: 1 in, 6 out]
            n977 = call <vilib>:"Add State(s) to Queue__JKI_lib_State_Machine.vi"("State(s) in Front (\"\")"="Set Vacuum Pump Speed" ("State(s) in Front (\"\")"), "State(s) in (\"\")"=w2953) -> ("States Out"=w2954:string)  [unwired: 13 in]
          }
        }
      }
      frame "---------- Core ----------" {
        # "Do not put any code in this frame.\n(it is a separator no-op)"
        n978 = call <vilib>:"Add State(s) to Queue__JKI_lib_State_Machine.vi"("State(s) in (\"\")"=w2963) -> ("States Out"=w2962:string)  [unwired: 14 in]
      }
      frame Default {
        w2975 = 42 items=["No error", "Argument error", "Memory is full", "Out of zone", "End of file", "File already open", "Generic file I/O error", "File not found", "File permission error", "Disk is full", "Duplicate path", "Too many files open", "System feature not enabled", "Resource file not found", "Cannot add resource", "Resource not found", "Image not found", "Image memory error", "Pen does not exist", "Config type invalid", "Config token not found", "Config parse error", "Config memory error", "Bad external code format", "Bad external code offset", "External code not present", "Null window", "Destroy window error", "Null menu", "Print aborted", "Bad print record", "Print driver error", "Windows error during printing", "Memory error during printing", "Print dialog error", "Generic print error", "Invalid device refnum", "Device not found", "Device parameter error", "Device unit error", "Cannot open device", "Device call aborted", "Generic error", "Cancelled by user", "Object ID too low", "Object ID too high", "Object not in heap", "Unknown heap", "Unknown object (invalid DefProc)", "Unknown object (DefProc not in table)", "Message out of range", "Invalid (null) method", "Unknown message", "Manager call not supported", "Bad address", "Network operation in progress", "Network operation timed out", "Connection is busy", "Network attribute not supported", "Network error", "Address in use", "System out of memory", "Connection aborted", "Connection refused", "Not connected", "Already connected", "Connection closed", "Initialization error (interapplication manager)", "Bad occurrence", "Wait on unbound occurrence handler", "Occurrence queue overflow", "Datalog type conflict", "Unused", "Unrecognized type (interapplication manager)", "Memory corrupt", "Failed to make temporary DLL", "Old CIN version", "Drag socket not found", "Failed to load drop-object", "Failed to register OLE object", "Failed to release OLE object", "Format specifier type mismatch", "Unknown format specifier", "Too few format specifiers", "Too many format specifiers", "Scan failed", "Newer CIN version", "Error converting to variant", "Runtime menu error", "Password tampered", "Variant attribute not found", "Incompatible variant data type", "Event data is not available", "Event Store is not present", "Occurrence is not found", "Event Queue is not created", "Event info is not available", "Refnum passed is NULL", "Error retrieving Class GUID", "Error retrieving CoClass GUID", "Error retrieving TypeLib GUID.", "Bad built application magic bytes.", "Specific driver is different from the specific driver associated with the Logical Name.", "There is no session opened to the class driver.", "Max Error", "MAX - Error with config objects", "MAX - Error loading configuration", "MAX - Group not supported"]
        # "Current State"
        # "Do not delete, rename, or modify this frame.\n(this is used to capture unhandled states and typos)"
        # "Handle mistyped state name (developer tool)"
        n979 = Format Into String(format string="Software Exception: Unhandled State \"%s\"." ("message"), error in=w2971, w2966) -> (resulting string=w2974:string, error out=w2973:errorcluster)  [unwired: 1 in]
        n980 = call <vilib>:"Error Cluster From Error Code.vi"("show call chain? (False)"=TRUE, "error in (no error)"=w2973, "error message (\"\")"=w2974, "error code (0)"=w2975) -> ("error out"=w2972:errorcluster)  [unwired: 5 in]
        n981 = call <vilib>:"Add State(s) to Queue__JKI_lib_State_Machine.vi"("State(s) in (\"\")"=w2970) -> ("States Out"=w2969:string)  [unwired: 14 in]
      }
      frame "Initialize Core Data" {
        # "Do not delete, rename, or modify this frame.\n(this is used to determine panel behavior on exit)"
        # "originally closed?"
        # "exe?"
        # "If panel starts closed or is an EXE, then close it when we exit"
        n982 = property class="VI"() -> ("Front Panel.Open"=w2986:bool)  [unwired: 2 in, 2 out]
        n983 = property class="App"() -> ("App.Kind"=w2985:T32)  [unwired: 2 in, 2 out]
        n984 = control-ref of="Current VI Reference"() -> (w2979:refnum<vi>)
        n985 = Not(x=w2986) -> (.not. x?=w2983:bool)
        n986 = Equal?(x=w2985, y=T32."Run Time System" ("Application:Kind")) -> (x = y?=w2982:bool)
        n987 = Or(x=w2983, y=w2982) -> (x .or. y?=w2980:bool)
        n988 = Bundle By Name(cluster=w2981, "Core.Current VI Reference"=w2979, "Core.Close Panel on Exit?"=w2980) -> (w2988:T77)
        n989 = call <vilib>:"Add State(s) to Queue__JKI_lib_State_Machine.vi"("State(s) in (\"\")"=w2990) -> ("States Out"=w2989:string)  [unwired: 14 in]
      }
      frame "Error Handler" {
        # "Unhandled Error -- Display it"
        # "Handle any errors here.\nYou can also output any states to clean-up after errors occur"
        # "Clear error"
        n990 = call <vilib>:"General Error Handler.vi"("error in (no error)"=w2994) -> ()  [unwired: 10 in, 5 out]
        n991 = call <vilib>:"Add State(s) to Queue__JKI_lib_State_Machine.vi"("State(s) in Front (\"\")"="/* Post Error States", "State(s) in (\"\")"=w2998) -> ("States Out"=w2997:string)  [unwired: 13 in]
      }
      frame "Exit" {
        # "Do not put any code in this frame.\n(No errors that occur here will be handled.)"
        n992 = call <vilib>:"Add State(s) to Queue__JKI_lib_State_Machine.vi"("State(s) in (\"\")"=w3005) -> ("States Out"=w3004:string)  [unwired: 14 in]
      }
      frame "---------- Data ----------" {
        n993 = call <vilib>:"Add State(s) to Queue__JKI_lib_State_Machine.vi"("State(s) in (\"\")"=w3011) -> ("States Out"=w3010:string)  [unwired: 14 in]
      }
      frame "Data: Read Head Status" {
        n994 = Unbundle By Name(w3019) -> ("GIS Printer"=w3018:refnum<class "GIS Printer.lvclass">)
        n995 = call "Read HeadStatus.vi"("error in (no error)"=w3017, "GIS Printer in"=w3018) -> ("error out"=w3013:errorcluster, "HeadStatus"=w3015:T71, "GIS Printer out"=w3014:refnum<class "GIS Printer.lvclass">)  [unwired: 7 in]
        n996 = call-dynamic "ForceHeadEnableStatus_GIS Printer.vi"("error in (no error)"=w3013, "GIS Printer In"=w3014) -> ("error out"=w3012:errorcluster)  [unwired: 8 in, 1 out]
        n997 = Bundle By Name(cluster=w3019, "HeadStatusPollData"=w3015) -> (w3016:T77)
        n998 = call <vilib>:"Add State(s) to Queue__JKI_lib_State_Machine.vi"("State(s) in (\"\")"=w3023) -> ("States Out"=w3022:string)  [unwired: 14 in]
      }
      frame "Data: Apply Init XML to UI" {
        n999 = call "FG - FilePathnames.vi"() -> ("FilePaths out"=w3031:T83)  [unwired: 4 in, 1 out]
        n1000 = Unbundle By Name(w3031) -> ("PrinterInitXMLFile"=w3030:path, "RecipeXMLFolder"=w3029:path, "CalibrationRecipeXMLFolder"=w3028:path)
        n1001 = property on="INITIALIZATION FILE PATH" class="Path"(error in=w3024, "Value"=w3030) -> (error out=w3027:errorcluster)  [unwired: 1 in, 1 out]
        n1002 = property on="PRODUCT RECIPE XML FOLDER PATH" class="Path"(error in=w3027, "Value"=w3029) -> (error out=w3026:errorcluster)  [unwired: 1 in, 1 out]
        n1003 = property on="CALIBRATION RECIPE XML FOLDER PATH" class="Path"(error in=w3026, "Value"=w3028) -> (error out=w3025:errorcluster)  [unwired: 1 in, 1 out]
        n1004 = call <vilib>:"Add State(s) to Queue__JKI_lib_State_Machine.vi"("State(s) in (\"\")"=w3036) -> ("States Out"=w3035:string)  [unwired: 14 in]
      }
      frame "Data: Update Pesrsistent Values" {
        n1005 = local read "Enable Ink Ch-1"() -> (w3049:bool)
        n1006 = local read "Enable Ink Ch-2"() -> (w3048:bool)
        n1007 = local read "Enable Ink Ch-3"() -> (w3047:bool)
        n1008 = local read "Enable Ink Ch-4"() -> (w3046:bool)
        n1009 = local read "Enable Ink Ch-5"() -> (w3045:bool)
        n1010 = local read "Enable Ink Ch-6"() -> (w3044:bool)
        n1011 = local read "Heater-1 Off 2"() -> (w3043:bool)
        n1012 = local read "Heater-2 Off 2"() -> (w3042:bool)
        n1013 = local read "Heater-3 Off 2"() -> (w3041:bool)
        n1014 = local read "Heater-4 Off 2"() -> (w3040:bool)
        n1015 = local read "Heater-5 Off 2"() -> (w3039:bool)
        n1016 = local read "Heater-6 Off 2"() -> (w3038:bool)
        n1017 = Bundle By Name(cluster=w3053, "PersistentData.InkChEnable.Enable Ink Ch-1"=w3049, "PersistentData.InkChEnable.Enable Ink Ch-2"=w3048, "PersistentData.InkChEnable.Enable Ink Ch-3"=w3047, "PersistentData.InkChEnable.Enable Ink Ch-4"=w3046, "PersistentData.InkChEnable.Enable Ink Ch-5"=w3045, "PersistentData.InkChEnable.Enable Ink Ch-6"=w3044, "PersistentData.HeatEnable.Heater-1 Off"=w3043, "PersistentData.HeatEnable.Heater-2 Off"=w3042, "PersistentData.HeatEnable.Heater-3 Off"=w3041, "PersistentData.HeatEnable.Heater-4 Off"=w3040, "PersistentData.HeatEnable.Heater-5 Off"=w3039, "PersistentData.HeatEnable.Heater-6 Off"=w3038) -> (w3050:T77)
        n1018 = call <vilib>:"Add State(s) to Queue__JKI_lib_State_Machine.vi"("State(s) in Front (\"\")"="Data: Write to Persistent File", "State(s) in (\"\")"=w3056) -> ("States Out"=w3055:string)  [unwired: 13 in]
      }
      frame "Data: Apply Persistent Data" {
        n1019 = Unbundle By Name(w3063) -> ("TopLevel out"=w3062:refnum<class "TopLevel.lvclass">, "PersistentData"=w3057:T72)
        n1020 = call "ApplyPersistentData.vi"("error in (no error)"=w3060, "PersistentData"=w3057, "TopLevel in"=w3062) -> ("error out"=w3061:errorcluster, "TopLevel out"=w3058:refnum<class "TopLevel.lvclass">)  [unwired: 7 in]
        n1021 = Bundle By Name(cluster=w3063, "TopLevel out"=w3058) -> (w3059:T77)
        n1022 = call <vilib>:"Add State(s) to Queue__JKI_lib_State_Machine.vi"("State(s) in (\"\")"=w3067) -> ("States Out"=w3066:string)  [unwired: 14 in]
      }
      frame "Data: Write to Persistent File" {
        n1023 = Unbundle By Name(w3072) -> ("TopLevel out"=w3071:refnum<class "TopLevel.lvclass">, "PersistentData"=w3068:T72)
        n1024 = call "FG - FilePathnames.vi"() -> ("FilePaths out"=w3073:T83)  [unwired: 4 in, 1 out]
        n1025 = Unbundle By Name(w3073) -> ("PersistentXMLFile"=w3074:path)
        n1026 = call-dynamic "Write PersistentXML.vi"("error in (no error)"=w3069, "PersistentData"=w3068, "TopLevel in"=w3071) -> ("error out"=w3075:errorcluster)  [unwired: 7 in, 1 out]
        n1027 = call "Persistent_XML_Write.vi"("error in (no error)"=w3075, "PersistentData"=w3068, "Persistent XML File Path"=w3074) -> ("error out"=w3070:errorcluster)  [unwired: 8 in]
      }
      frame "Data: LoadRecipe" {
        w3092 = T68 {"Path"=path "", "Type"="", "Product"=""} ("RecipeInfo")
        # "This state loads the selected print recipe"
        n1028 = Unbundle By Name(w3084) -> ("Methods:Accessors:ConfigDict"=w3090:T16)
        n1029 = call <vilib>:"Get Dynamic CVT Data.vi"("error in (no error)"=w3087, "default value (empty variant)"=w3092, "DataName"=w3086, "dCVT DVR"=w3090) -> ("error out"=w3094:errorcluster, "value"=w3093:variant)  [unwired: 4 in, 2 out]
        n1030 = Variant To Data(error in=w3094, type=w3092, Variant=w3093) -> (data=w3082:T68, error out=w3089:errorcluster)
        n1031 = Unbundle By Name(w3082) -> ("Path"=w3083:path, "Type"=w3091:string)
        "Type" <- w3091
        n1032 = case shown="\"Calibration\"" w3091 {
          tunnel: w3083 -> [_ w3103 w3107]
          tunnel: w3089 -> [w3099 w3102 w3106]
          tunnel: [w3099 w3101 w3105] -> w3088
          tunnel: [_ w3100 _] -> w3081
          tunnel: [_ _ w3104] -> w3079
          frame Default {
          }
          frame "PrintDesign" {
            n1033 = call "DLP_RecipePrints_XML_Read.vi"("error in (no error)"=w3102, "Recipe XML File Path"=w3103) -> ("error out"=w3101:errorcluster, "DLPRecipe"=w3100:T73)  [unwired: 8 in]
          }
          frame "Calibration" {
            n1034 = call "DLP_CalibrationPrints_XML_Read.vi"("error in (no error)"=w3106, "Recipe XML File Path"=w3107) -> ("error out"=w3105:errorcluster, "CalibrationPrints"=w3104:T74)  [unwired: 8 in]
          }
        }
        n1035 = Bundle By Name(cluster=w3084, "PrintDesign"=w3082, "CurrentDLPRecipe"=w3081, "CalibrationPrints"=w3079) -> (w3085:T77)
        n1036 = call <vilib>:"Add State(s) to Queue__JKI_lib_State_Machine.vi"("State(s) in Front (\"\")"="" ("State(s) in Front (\"\")"), "State(s) in (\"\")"=w3098) -> ("States Out"=w3097:string)  [unwired: 13 in]
      }
      frame "Data: GetProductRecipeNames" {
        w3117 = T84 {"Product"="", "RecipePathsByProduct"=[], "RecipeNamesByProduct"=[]}
        n1037 = Unbundle By Name(w3115) -> ("Methods:Accessors:ConfigDict"=w3114:T16)
        n1038 = call <vilib>:"Get Dynamic CVT Data.vi"("error in (no error)"=w3110, "default value (empty variant)"=w3117, "DataName"=w3109, "dCVT DVR"=w3114) -> ("error out"=w3119:errorcluster, "value"=w3118:variant)  [unwired: 4 in, 2 out]
        n1039 = Variant To Data(error in=w3119, type=w3117, Variant=w3118) -> (data=w3116:T84, error out=w3112:errorcluster)
        n1040 = Unbundle By Name(w3116) -> ("RecipeNamesByProduct"=w3113:string[])
        n1041 = property on="Recipe" class="Ring (strict)"(error in=w3112, "Strings []"=w3113, "Val(Sgnl)"=0) -> (error out=w3111:errorcluster)  [unwired: 1 in, 1 out]
        n1042 = call <vilib>:"Add State(s) to Queue__JKI_lib_State_Machine.vi"("State(s) in (\"\")"=w3123) -> ("States Out"=w3122:string)  [unwired: 14 in]
      }
      frame "Data: Populate Products" {
        w3131 = string[] [] ("elements")
        n1043 = Unbundle By Name(w3129) -> ("Methods:Accessors:ConfigDict"=w3136:T16)
        n1044 = Concatenate Strings(w3130, "Products" ("string")) -> (w3134:string)
        n1045 = call <vilib>:"Get Dynamic CVT Data.vi"("error in (no error)"=w3125, "default value (empty variant)"=w3131, "DataName"=w3134, "dCVT DVR"=w3136) -> ("error out"=w3133:errorcluster, "value"=w3132:variant)  [unwired: 4 in, 2 out]
        n1046 = Variant To Data(error in=w3133, type=w3131, Variant=w3132) -> (data=w3128:string[], error out=w3127:errorcluster)
        n1047 = property on="Product" class="Ring (strict)"(error in=w3127, "Strings []"=w3128, "Val(Sgnl)"=0) -> (error out=w3126:errorcluster)  [unwired: 1 in, 1 out]
        n1048 = call <vilib>:"Add State(s) to Queue__JKI_lib_State_Machine.vi"("State(s) in (\"\")"=w3140) -> ("States Out"=w3139:string)  [unwired: 14 in]
      }
      frame "UpdateSettings" {
        n1049 = Unbundle By Name(w3142) -> ("SettingsUpdate"=w3141:variant)
        n1050 = Concatenate Strings("UpdateSettings>>" ("states in"), w3148) -> (w3146:string)
        n1051 = call <vilib>:"Add State to Queue with vData.vi"("queue in"=w3145, "state in"=w3146, "vData (\"\")"=w3141, "error in"=w3143) -> ("error out"=w3144:errorcluster)  [unwired: 8 in, 3 out]
        n1052 = call <vilib>:"Add State(s) to Queue__JKI_lib_State_Machine.vi"("State(s) in (\"\")"=w3152) -> ("States Out"=w3151:string)  [unwired: 14 in]
      }
      frame "Data: Verify Materials and Color planes" {
        n1053 = disable-structure shown="Disabled" {
          disable-tunnel: w3153 -> [w3179 _]
          frame Disabled {
